vi "New.vi"(8 "error in (no error)":errorcluster, 11 "ChannelMap":map{T1, refnum<data-value>}(c390)) -> (0 "error out":errorcluster, 2 "callback UEs":T2, 3 "BluePlotHandleDemo out":refnum<class "BluePlotHandleDemo.lvclass">)   [LabVIEW 2021, in "BluePlotDemo.lvlib" / "BluePlotHandleDemo.lvclass"]
uses:
  BluePlotHandleDemo.lvclass
  BluePlotHandleDemo.lvclass/BluePlotHandleDemo.ctl
  SubVIs/Demo Names.ctl
  BluePlotDemo.lvlib
  <vilib>/National Instruments/Variant Ring Buffer/Ring Buffer.lvclass
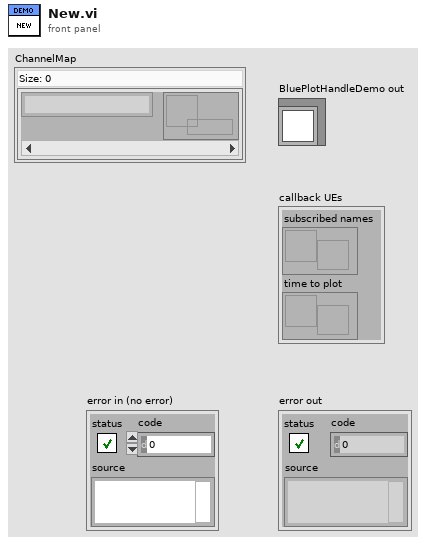
[diagram p1: front panel]
types:
  T1 = typedef "BluePlotDemo.lvlib/Demo Names.ctl" = enum16{"Sine Wave", "Triangle Wave", "Sawtooth Wave", "Square Wave", "Uniform Noise", "Periodic Noise", "White Noise"}
  T2 = cluster{"subscribed names":refnum<user-event>, "time to plot":refnum<user-event>}
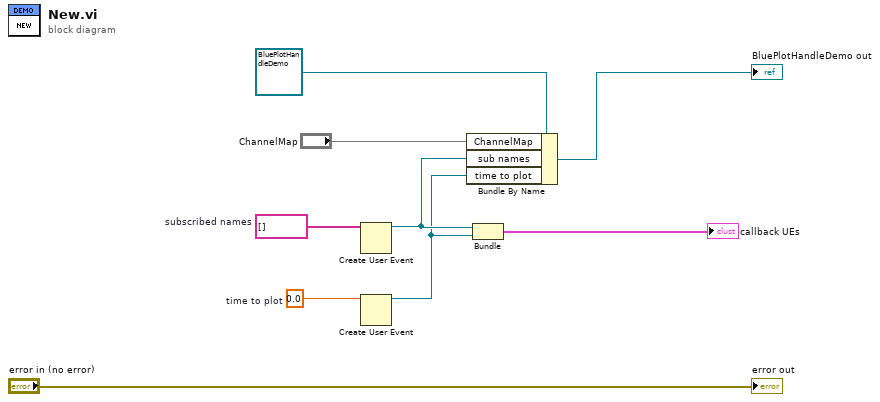
[diagram p0: block diagram]
diagram:
  w5 = 0.0  # time to plot
  w8 = string[] []  # subscribed names
  n1 = Create User Event(user event datatype=w8) -> (user event=w4:refnum<user-event>)  [unwired: 1 in, 1 out]
  n2 = Create User Event(user event datatype=w5) -> (user event=w3:refnum<user-event>)  [unwired: 1 in, 1 out]
  n3 = Bundle By Name(cluster=refnum<class "BluePlotHandleDemo.lvclass"> refnum ("BluePlotHandleDemo out"), "ChannelMap"="ChannelMap", "sub names"=w4, "time to plot"=w3) -> (→"BluePlotHandleDemo out":refnum<class "BluePlotHandleDemo.lvclass">)
  n4 = Bundle("subscribed names"=w4, "time to plot"=w3) -> (→"callback UEs":T2)  [unwired: 1 in]
  "error out" <- "error in (no error)"
